vi "Abstract LV Class - Hierarchy.vi"   [LabVIEW 2021]
uses:
  Abs_Types/Type/Abs_Type.lvclass
  Abs_Types/Value/Abs_Value.lvclass
  Abs_Types/Numeric/Abs_Numeric.lvclass
  Abs_Types/Floating Point/Abs_Floating Point.lvclass
  Abs_Types/Single Float/Abs_Single Float.lvclass
  Abs_Types/Double Float/Abs_Double Float.lvclass
  Abs_Types/Extended Float/Abs_Extended Float.lvclass
  Abs_Types/Complex Double Float/Abs_Complex Double Float.lvclass
  Abs_Types/Complex Extended Float/Abs_Complex Extended Float.lvclass
  Abs_Types/Complex Single Float/Abs_Complex Single Float.lvclass
  Abs_Types/Integer/Abs_Integer.lvclass
  Abs_Types/I8 Integer/Abs_I8 Integer.lvclass
  Abs_Types/I16 Integer/Abs_I16 Integer.lvclass
  Abs_Types/I32 Integer/Abs_I32 Integer.lvclass
  Abs_Types/I64 Integer/Abs_I64 Integer.lvclass
  Abs_Types/U8 Integer/Abs_U8 Integer.lvclass
  Abs_Types/U16 Integer/Abs_U16 Integer.lvclass
  Abs_Types/U32 Integer/Abs_U32 Integer.lvclass
  Abs_Types/U64 Integer/Abs_U64 Integer.lvclass
  Abs_Types/Time/Abs_Time.lvclass
  Abs_Types/Boolean/Abs_Boolean.lvclass
  Abs_Types/String/Abs_String.lvclass
  Abs_Types/Variant/Abs_Variant.lvclass
  Abs_Types/Waveform/Abs_Waveform.lvclass
  Abs_Types/Boolean/Static Write.vi
  Abs_Types/Double Float/Simple Read.vi
  Abs_Types/Boolean/Static Read.vi
panel:
  # "SEE DIAGRAM\nFOR Hierarchy"
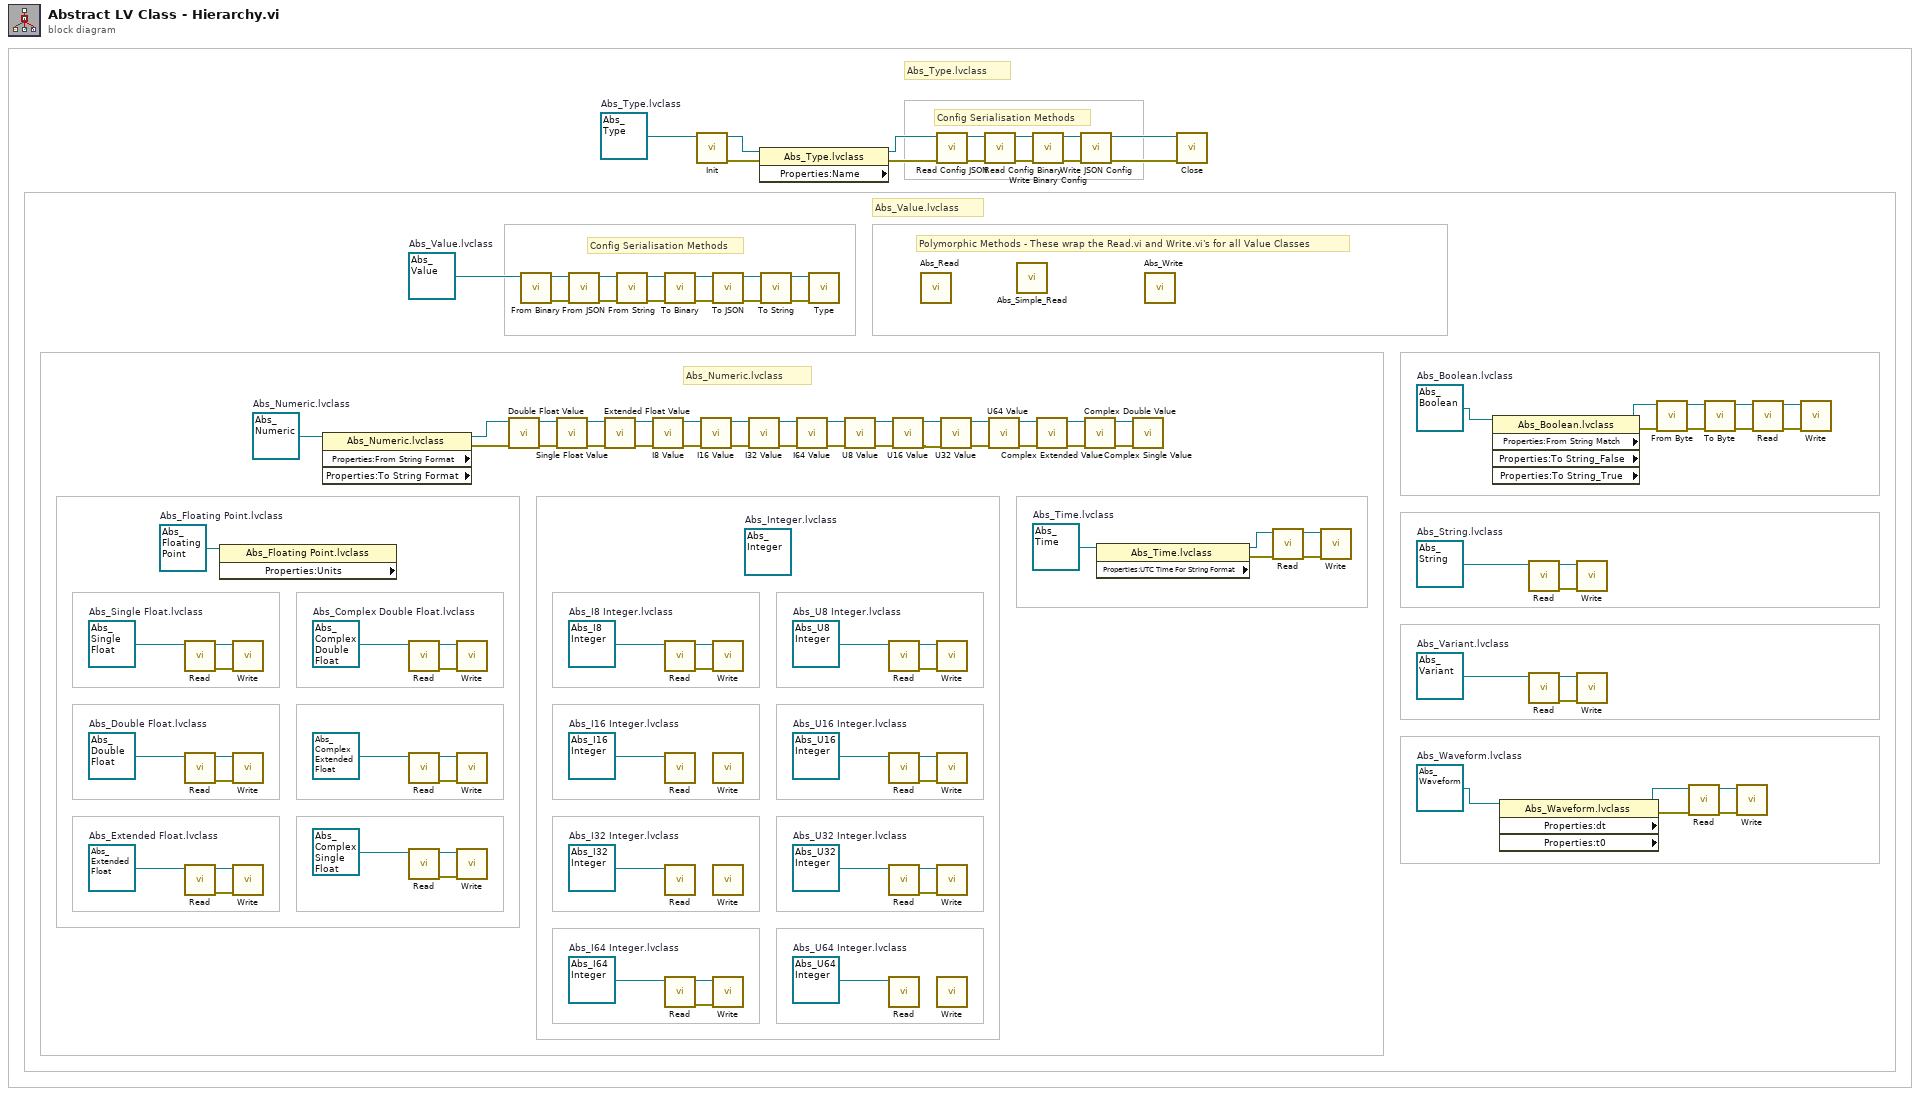
[diagram p0: block diagram]
diagram:
  w5 = refnum<class "Abs_Waveform.lvclass"> refnum  # Abs_Waveform.lvclass
  w6 = refnum<class "Abs_Variant.lvclass"> refnum  # Abs_Variant.lvclass
  w11 = refnum<class "Abs_String.lvclass"> refnum  # Abs_String.lvclass
  w20 = refnum<class "Abs_Boolean.lvclass"> refnum  # Abs_Boolean.lvclass
  w25 = refnum<class "Abs_Time.lvclass"> refnum  # Abs_Time.lvclass
  w35 = refnum<class "Abs_U64 Integer.lvclass"> refnum  # Abs_U64 Integer.lvclass
  w34 = refnum<class "Abs_U32 Integer.lvclass"> refnum  # Abs_U32 Integer.lvclass
  w32 = refnum<class "Abs_U16 Integer.lvclass"> refnum  # Abs_U16 Integer.lvclass
  w33 = refnum<class "Abs_U8 Integer.lvclass"> refnum  # Abs_U8 Integer.lvclass
  w38 = refnum<class "Abs_I64 Integer.lvclass"> refnum  # Abs_I64 Integer.lvclass
  w37 = refnum<class "Abs_I32 Integer.lvclass"> refnum  # Abs_I32 Integer.lvclass
  w36 = refnum<class "Abs_I16 Integer.lvclass"> refnum  # Abs_I16 Integer.lvclass
  w43 = refnum<class "Abs_I8 Integer.lvclass"> refnum  # Abs_I8 Integer.lvclass
  (unwired) refnum<class "Abs_Integer.lvclass"> refnum  # Abs_Integer.lvclass
  w52 = refnum<class "Abs_Complex Double Float.lvclass"> refnum  # Abs_Complex Double Float.lvclass
  w55 = refnum<class "Abs_Extended Float.lvclass"> refnum  # Abs_Extended Float.lvclass
  w58 = refnum<class "Abs_Double Float.lvclass"> refnum  # Abs_Double Float.lvclass
  w61 = refnum<class "Abs_Single Float.lvclass"> refnum  # Abs_Single Float.lvclass
  w62 = refnum<class "Abs_Floating Point.lvclass"> refnum  # Abs_Floating Point.lvclass
  w91 = refnum<class "Abs_Numeric.lvclass"> refnum  # Abs_Numeric.lvclass
  w104 = refnum<class "Abs_Value.lvclass"> refnum  # Abs_Value.lvclass
  w117 = refnum<class "Abs_Type.lvclass"> refnum  # Abs_Type.lvclass
  # "Abs_Numeric.lvclass"
  # "Polymorphic Methods - These wrap the Read.vi and Write.vi's for all Value Classes"
  # "Config Serialisation Methods"
  # "Abs_Value.lvclass"
  # "Abs_Type.lvclass"
  # "Config Serialisation Methods"
  n1 = call-dynamic "Read.vi"("Double Float.lvclass_340760 in"=w61) -> ("error out"=w59:errorcluster, "Double Float.lvclass_340760 out"=w60:refnum<class "Abs_Single Float.lvclass">)  [unwired: 8 in, 1 out]
  n2 = call-dynamic "Read.vi"("Double Float.lvclass_340760 in"=w58) -> ("error out"=w56:errorcluster, "Double Float.lvclass_340760 out"=w57:refnum<class "Abs_Double Float.lvclass">)  [unwired: 8 in, 1 out]
  n3 = call-dynamic "Read.vi"("Double Float.lvclass_340760 in"=w55) -> ("error out"=w53:errorcluster, "Double Float.lvclass_340760 out"=w54:refnum<class "Abs_Extended Float.lvclass">)  [unwired: 8 in, 1 out]
  n4 = property class="Abs_Floating Point.lvclass" props=["Properties:Units"](reference=w62) -> ()  [unwired: 1 in, 3 out]
  n5 = call-dynamic "Write.vi"("error in (no error)"=w59, "Double Float.lvclass_340760 in"=w60) -> ()  [unwired: 8 in, 2 out]
  n6 = call-dynamic "Write.vi"("error in (no error)"=w56, "Double Float.lvclass_340760 in"=w57) -> ()  [unwired: 8 in, 2 out]
  n7 = call-dynamic "Write.vi"("error in (no error)"=w53, "Double Float.lvclass_340760 in"=w54) -> ()  [unwired: 8 in, 2 out]
  n8 = property class="Abs_Numeric.lvclass" props=["Properties:From String Format", "Properties:To String Format"](reference=w91) -> (reference out=w89:refnum<class "Abs_Numeric.lvclass">, error out=w90:errorcluster)  [unwired: 1 in, 2 out]
  n9 = call-dynamic "Read.vi"("Double Float.lvclass_340760 in"=w52) -> ("error out"=w50:errorcluster, "Double Float.lvclass_340760 out"=w51:refnum<class "Abs_Complex Double Float.lvclass">)  [unwired: 8 in, 1 out]
  n10 = call-dynamic "Read.vi"("Double Float.lvclass_340760 in"=refnum<class "Abs_Complex Extended Float.lvclass"> refnum ("Abs_Complex Extended Float.lvclass")) -> ("error out"=w47:errorcluster, "Double Float.lvclass_340760 out"=w48:refnum<class "Abs_Complex Extended Float.lvclass">)  [unwired: 8 in, 1 out]
  n11 = call-dynamic "Read.vi"("Double Float.lvclass_340760 in"=refnum<class "Abs_Complex Single Float.lvclass"> refnum ("Abs_Complex Single Float.lvclass")) -> ("error out"=w44:errorcluster, "Double Float.lvclass_340760 out"=w45:refnum<class "Abs_Complex Single Float.lvclass">)  [unwired: 8 in, 1 out]
  n12 = call-dynamic "Write.vi"("error in (no error)"=w50, "Double Float.lvclass_340760 in"=w51) -> ()  [unwired: 8 in, 2 out]
  n13 = call-dynamic "Write.vi"("error in (no error)"=w47, "Double Float.lvclass_340760 in"=w48) -> ()  [unwired: 8 in, 2 out]
  n14 = call-dynamic "Write.vi"("error in (no error)"=w44, "Double Float.lvclass_340760 in"=w45) -> ()  [unwired: 8 in, 2 out]
  n15 = call-dynamic "Double Float Value.vi"("error in (no error)"=w90, "Numeric in"=w89) -> ("error out"=w79:errorcluster, "Numeric out"=w88:refnum<class "Abs_Numeric.lvclass">)  [unwired: 7 in, 1 out]
  n16 = call-dynamic "From Binary.vi"("Type in"=w104) -> ("error out"=w97:errorcluster, "Type out"=w103:refnum<class "Abs_Value.lvclass">)  [unwired: 8 in, 1 out]
  n17 = call-dynamic "Single Float Value.vi"("error in (no error)"=w79, "Numeric in"=w88) -> ("error out"=w78:errorcluster, "Numeric out"=w87:refnum<class "Abs_Numeric.lvclass">)  [unwired: 7 in, 1 out]
  n18 = call-dynamic "From JSON.vi"("error in (no error)"=w97, "Type in"=w103) -> ("error out"=w96:errorcluster, "Type out"=w102:refnum<class "Abs_Value.lvclass">)  [unwired: 8 in]
  n19 = call-dynamic "Extended Float Value.vi"("error in (no error)"=w78, "Numeric in"=w87) -> ("error out"=w77:errorcluster, "Numeric out"=w86:refnum<class "Abs_Numeric.lvclass">)  [unwired: 7 in, 1 out]
  n20 = call-dynamic "From String.vi"("error in (no error)"=w96, "Type in"=w102) -> ("error out"=w95:errorcluster, "Type out"=w101:refnum<class "Abs_Value.lvclass">)  [unwired: 6 in, 2 out]
  n21 = call-dynamic "I8 Value.vi"("error in (no error)"=w77, "Numeric in"=w86) -> ("error out"=w76:errorcluster, "Numeric out"=w85:refnum<class "Abs_Numeric.lvclass">)  [unwired: 7 in, 1 out]
  n22 = call-dynamic "To Binary.vi"("error in (no error)"=w95, "Type in"=w101) -> ("error out"=w94:errorcluster, "Type out"=w100:refnum<class "Abs_Value.lvclass">)  [unwired: 7 in, 1 out]
  n23 = call-dynamic "Read.vi"("Double Float.lvclass_340760 in"=w43) -> ("error out"=w41:errorcluster, "Double Float.lvclass_340760 out"=w42:refnum<class "Abs_I8 Integer.lvclass">)  [unwired: 8 in, 1 out]
  n24 = call-dynamic "Read.vi"("Double Float.lvclass_340760 in"=w36) -> ()  [unwired: 8 in, 3 out]
  n25 = call-dynamic "Read.vi"("Double Float.lvclass_340760 in"=w37) -> ()  [unwired: 8 in, 3 out]
  n26 = call-dynamic "Read.vi"("Double Float.lvclass_340760 in"=w38) -> ("error out"=w39:errorcluster, "Double Float.lvclass_340760 out"=w40:refnum<class "Abs_I64 Integer.lvclass">)  [unwired: 8 in, 1 out]
  n27 = call-dynamic "Init.vi"("Data in"=w117) -> ("error out"=w116:errorcluster, "Data out"=w115:refnum<class "Abs_Type.lvclass">)  [unwired: 9 in]
  n28 = call-dynamic "I16 Value.vi"("error in (no error)"=w76, "Numeric in"=w85) -> ("error out"=w75:errorcluster, "Numeric out"=w84:refnum<class "Abs_Numeric.lvclass">)  [unwired: 7 in, 1 out]
  n29 = call-dynamic "To JSON.vi"("error in (no error)"=w94, "Type in"=w100) -> ("error out"=w93:errorcluster, "Type out"=w99:refnum<class "Abs_Value.lvclass">)  [unwired: 7 in, 1 out]
  n30 = call-dynamic "Write.vi"("error in (no error)"=w41, "Double Float.lvclass_340760 in"=w42) -> ()  [unwired: 8 in, 2 out]
  n31 = call-dynamic "Write.vi"() -> ()  [unwired: 10 in, 2 out]
  n32 = call-dynamic "Write.vi"() -> ()  [unwired: 10 in, 2 out]
  n33 = call-dynamic "Write.vi"("error in (no error)"=w39, "Double Float.lvclass_340760 in"=w40) -> ()  [unwired: 8 in, 2 out]
  n34 = call-dynamic "I32 Value.vi"("error in (no error)"=w75, "Numeric in"=w84) -> ("error out"=w74:errorcluster, "Numeric out"=w83:refnum<class "Abs_Numeric.lvclass">)  [unwired: 7 in, 1 out]
  n35 = property class="Abs_Type.lvclass" props=["Properties:Name"](reference=w115, error in=w116) -> (reference out=w113:refnum<class "Abs_Type.lvclass">, error out=w114:errorcluster)  [unwired: 1 out]
  n36 = call-dynamic "To String.vi"("error in (no error)"=w93, "Types in"=w99) -> ("error out"=w92:errorcluster, "Types out"=w98:refnum<class "Abs_Value.lvclass">)  [unwired: 7 in, 1 out]
  n37 = call-dynamic "I64 Value.vi"("error in (no error)"=w74, "Numeric in"=w83) -> ("error out"=w73:errorcluster, "Numeric out"=w82:refnum<class "Abs_Numeric.lvclass">)  [unwired: 7 in, 1 out]
  n38 = call-dynamic "Type.vi"("error in (no error)"=w92, "Element in"=w98) -> ()  [unwired: 7 in, 3 out]
  n39 = call-dynamic "U8 Value.vi"("error in (no error)"=w73, "Numeric in"=w82) -> ("error out"=w72:errorcluster, "Numeric out"=w81:refnum<class "Abs_Numeric.lvclass">)  [unwired: 7 in, 1 out]
  n40 = call-dynamic "Read.vi"("Double Float.lvclass_340760 in"=w33) -> ("error out"=w30:errorcluster, "Double Float.lvclass_340760 out"=w31:refnum<class "Abs_U8 Integer.lvclass">)  [unwired: 8 in, 1 out]
  n41 = call-dynamic "Read.vi"("Double Float.lvclass_340760 in"=w32) -> ("error out"=w28:errorcluster, "Double Float.lvclass_340760 out"=w29:refnum<class "Abs_U16 Integer.lvclass">)  [unwired: 8 in, 1 out]
  n42 = call-dynamic "Read.vi"("Double Float.lvclass_340760 in"=w34) -> ("error out"=w26:errorcluster, "Double Float.lvclass_340760 out"=w27:refnum<class "Abs_U32 Integer.lvclass">)  [unwired: 8 in, 1 out]
  n43 = call-dynamic "Read.vi"("Double Float.lvclass_340760 in"=w35) -> ()  [unwired: 8 in, 3 out]
  n44 = call-dynamic "U16 Value.vi"("error in (no error)"=w72, "Numeric in"=w81) -> ("error out"=w71:errorcluster, "Numeric out"=w80:refnum<class "Abs_Numeric.lvclass">)  [unwired: 7 in, 1 out]
  n45 = call-poly "Abs_Read.vi"() -> ()  [unwired: 9 in, 3 out]
  n46 = call "Read Config JSON.vi"("error in (no error)"=w114, "Abs_Type in"=w113) -> ("error out"=w112:errorcluster, "Abs_Type out"=w111:refnum<class "Abs_Type.lvclass">)  [unwired: 8 in]
  n47 = call-dynamic "Write.vi"("error in (no error)"=w30, "Double Float.lvclass_340760 in"=w31) -> ()  [unwired: 8 in, 2 out]
  n48 = call-dynamic "Write.vi"("error in (no error)"=w28, "Double Float.lvclass_340760 in"=w29) -> ()  [unwired: 8 in, 2 out]
  n49 = call-dynamic "Write.vi"("error in (no error)"=w26, "Double Float.lvclass_340760 in"=w27) -> ()  [unwired: 8 in, 2 out]
  n50 = call-dynamic "Write.vi"() -> ()  [unwired: 10 in, 2 out]
  n51 = call-dynamic "U32 Value.vi"("error in (no error)"=w71, "Numeric in"=w80) -> ("error out"=w70:errorcluster, "Numeric out"=w69:refnum<class "Abs_Numeric.lvclass">)  [unwired: 7 in, 1 out]
  n52 = call "Read Config Binary.vi"("error in (no error)"=w112, "Abs_Type in"=w111) -> ("error out"=w110:errorcluster, "Abs_Type out"=w109:refnum<class "Abs_Type.lvclass">)  [unwired: 7 in, 1 out]
  n53 = call-dynamic "U64 Value.vi"("error in (no error)"=w70, "Numeric in"=w69) -> ("error out"=w67:errorcluster, "Numeric out"=w68:refnum<class "Abs_Numeric.lvclass">)  [unwired: 7 in, 1 out]
  n54 = call-poly "Abs_Simple_Read.vi"() -> ()  [unwired: 5 in, 1 out]
  n55 = call-dynamic "Write Binary Config.vi"("error in (no error)"=w110, "Abs_Type in"=w109) -> ("error out"=w107:errorcluster, "Abs_Type out"=w108:refnum<class "Abs_Type.lvclass">)  [unwired: 7 in, 1 out]
  n56 = call-dynamic "Complex Extended Value.vi"("error in (no error)"=w67, "Numeric in"=w68) -> ("error out"=w66:errorcluster, "Numeric out"=w65:refnum<class "Abs_Numeric.lvclass">)  [unwired: 7 in, 1 out]
  n57 = call-dynamic "Write JSON Config.vi"("error in (no error)"=w107, "Abs_Type in"=w108) -> ("error out"=w106:errorcluster, "Abs_Type out"=w105:refnum<class "Abs_Type.lvclass">)  [unwired: 7 in, 1 out]
  n58 = call-dynamic "Complex Double Value.vi"("error in (no error)"=w66, "Numeric in"=w65) -> ("error out"=w63:errorcluster, "Numeric out"=w64:refnum<class "Abs_Numeric.lvclass">)  [unwired: 7 in, 1 out]
  n59 = property class="Abs_Time.lvclass" props=["Properties:UTC Time For String Format"](reference=w25) -> (reference out=w21:refnum<class "Abs_Time.lvclass">, error out=w24:errorcluster)  [unwired: 1 in, 1 out]
  n60 = call-dynamic "Complex Single Value.vi"("error in (no error)"=w63, "Numeric in"=w64) -> ()  [unwired: 7 in, 3 out]
  n61 = call-poly "Abs_Write.vi"() -> ()  [unwired: 10 in, 2 out]
  n62 = call-dynamic "Close.vi"("error in (no error)"=w106, "Data in"=w105) -> ()  [unwired: 8 in, 2 out]
  n63 = call-dynamic "Read.vi"("error in (no error)"=w24, "Double Float.lvclass_340760 in"=w21) -> ("error out"=w23:errorcluster, "Double Float.lvclass_340760 out"=w22:refnum<class "Abs_Time.lvclass">)  [unwired: 7 in, 1 out]
  n64 = call-dynamic "Write.vi"("error in (no error)"=w23, "Double Float.lvclass_340760 in"=w22) -> ()  [unwired: 8 in, 2 out]
  n65 = property class="Abs_Boolean.lvclass" props=["Properties:From String Match", "Properties:To String_False", "Properties:To String_True"](reference=w20) -> (reference out=w18:refnum<class "Abs_Boolean.lvclass">, error out=w19:errorcluster)  [unwired: 1 in, 3 out]
  n66 = property class="Abs_Waveform.lvclass" props=["Properties:dt", "Properties:t0"](reference=w5) -> (reference out=w4:refnum<class "Abs_Waveform.lvclass">, error out=w3:errorcluster)  [unwired: 1 in, 2 out]
  n67 = call-dynamic "Read.vi"("Abs_String in"=w11) -> ("error out"=w9:errorcluster, "Abs_String out"=w10:refnum<class "Abs_String.lvclass">)  [unwired: 8 in, 1 out]
  n68 = call-dynamic "Read.vi"("Abs_Variant in"=w6) -> ("error out"=w7:errorcluster, "Abs_Variant out"=w8:refnum<class "Abs_Variant.lvclass">)  [unwired: 8 in, 1 out]
  n69 = call-dynamic "Write.vi"("error in (no error)"=w9, "Abs_String in"=w10) -> ()  [unwired: 8 in, 2 out]
  n70 = call-dynamic "Write.vi"("error in (no error)"=w7, "Abs_Variant in"=w8) -> ()  [unwired: 8 in, 2 out]
  n71 = call-dynamic "From Byte.vi"("error in (no error)"=w19, "Boolean in"=w18) -> ("error out"=w16:errorcluster, "Boolean out"=w17:refnum<class "Abs_Boolean.lvclass">)  [unwired: 8 in]
  n72 = call-dynamic "Read.vi"("error in (no error)"=w3, "Abs_Waveform in"=w4) -> ("error out"=w2:errorcluster, "Abs_Waveform out"=w1:refnum<class "Abs_Waveform.lvclass">)  [unwired: 7 in, 1 out]
  n73 = call-dynamic "To Byte.vi"("error in (no error)"=w16, "Boolean in"=w17) -> ("error out"=w14:errorcluster, "Boolean out"=w15:refnum<class "Abs_Boolean.lvclass">)  [unwired: 8 in]
  n74 = call-dynamic "Write.vi"("error in (no error)"=w2, "Abs_Waveform in"=w1) -> ()  [unwired: 8 in, 2 out]
  n75 = call-dynamic "Read.vi"("error in (no error)"=w14, "Boolean in"=w15) -> ("error out"=w12:errorcluster, "Boolean out"=w13:refnum<class "Abs_Boolean.lvclass">)  [unwired: 7 in, 1 out]
  n76 = call-dynamic "Write.vi"("error in (no error)"=w12, "Boolean in"=w13) -> ()  [unwired: 8 in, 2 out]
